vi "AppenderConfigFromDTO.vi"(8 "error in (no error)":errorcluster, 11 "AppenderConfigDTO":T6={"id"="", "threshold"="INFO", "filter"={"mode"="Mirror", "levelMin"="INFO", "levelMax"="INFO", "tagPrefix"=""}, "queueBound"=0, "dropPolicy"="DropOldest", "useUTC"=FALSE}) -> (0 "error out":errorcluster, 3 "AppenderConfig":T1={"id"="", "threshold"=enum."INFO", "filter"={"mode"=enum."Mirror", "levelMin"=enum."INFO", "levelMax"=enum."INFO", "tagPrefix"=""}, "queueBound"=0, "dropPolicy"=enum."DropOldest", "useUTC"=FALSE})   [LabVIEW 2026, in "Lumberjack.lvlib"]
uses:
  Lumberjack.lvlib
  TypeDefs/ConfigDTO/AppenderConfigDTO.ctl
  TypeDefs/ConfigDTO/FilterDTO.ctl
  TypeDefs/AppenderConfig.ctl
  TypeDefs/Severity.ctl
  TypeDefs/Filter.ctl
  TypeDefs/FilterMode.ctl
  TypeDefs/DropPolicy.ctl
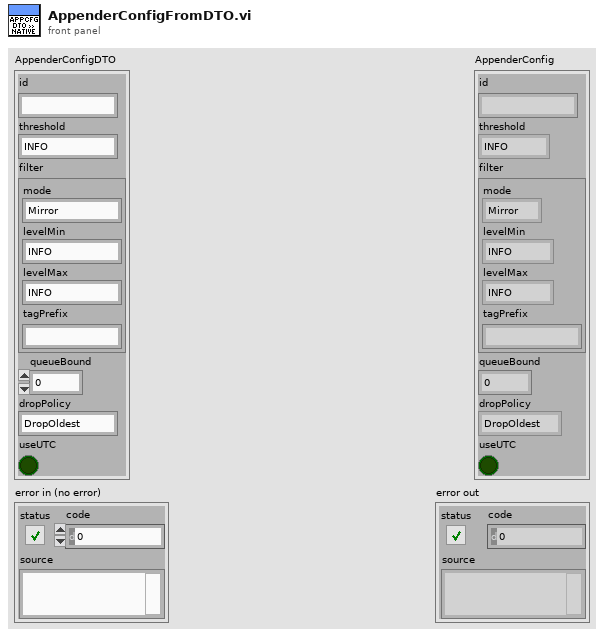
[diagram p1: front panel]
types:
  T1 = typedef "Lumberjack.lvlib/AppenderConfig.ctl" = cluster{"id":string, "threshold":T2, "filter":T3, "queueBound":i32, "dropPolicy":T5, "useUTC":bool}
  T2 = typedef "Lumberjack.lvlib/Severity.ctl" = enum16{"OFF", "FATAL", "ERROR", "WARN", "INFO", "DEBUG", "TRACE", "ALL"}
  T3 = typedef "Lumberjack.lvlib/Filter.ctl" = cluster{"mode":T4, "levelMin":T2, "levelMax":T2, "tagPrefix":string}
  T4 = typedef "Lumberjack.lvlib/FilterMode.ctl" = enum16{"Mirror", "Routed"}
  T5 = typedef "Lumberjack.lvlib/DropPolicy.ctl" = enum16{"DropOldest", "DropNewest", "LevelAware"}
  T6 = typedef "Lumberjack.lvlib/AppenderConfigDTO.ctl" = cluster{"id":string, "threshold":string, "filter":T7, "queueBound":i32, "dropPolicy":string, "useUTC":bool}
  T7 = typedef "Lumberjack.lvlib/FilterDTO.ctl" = cluster{"mode":string, "levelMin":string, "levelMax":string, "tagPrefix":string}
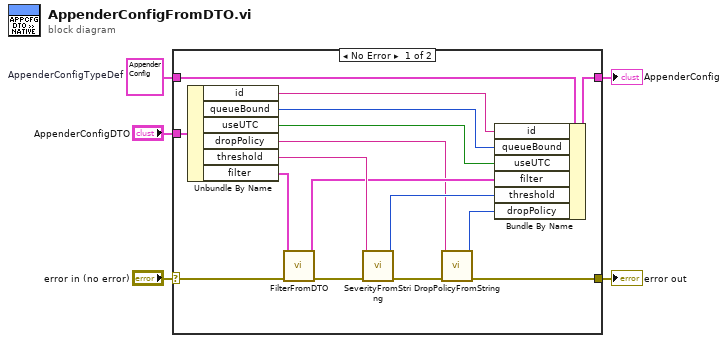
[diagram p0: block diagram]
diagram:
  w2 = T1 {"id"="", "threshold"=enum."INFO", "filter"={"mode"=enum."Mirror", "levelMin"=enum."INFO", "levelMax"=enum."INFO", "tagPrefix"=""}, "queueBound"=0, "dropPolicy"=enum."DropOldest", "useUTC"=FALSE}  # AppenderConfigTypeDef
  n1 = case shown="No Error" "error in (no error)" {
    selector: "error in (no error)" -> [w21 w23]
    tunnel: [w18 w23] -> w4
    tunnel: "AppenderConfigDTO" -> [w16 _]
    tunnel: w2 -> [w15 w22]
    tunnel: [w17 w22] -> w3
    frame No Error {
      n2 = Unbundle By Name(w16) -> ("id"=w14:string, "queueBound"=w13:i32, "useUTC"=w6:bool, "dropPolicy"=w7:string, "threshold"=w11:string, "filter"=w12:T7)
      n3 = call "FilterFromDTO.vi"("error in (no error)"=w21, "FilterDTO"=w12) -> ("error out"=w20:errorcluster, "Filter"=w8:T3)  [unwired: 8 in]
      n4 = call "SeverityFromString.vi"("error in (no error)"=w20, "SeverityString"=w11) -> ("error out"=w19:errorcluster, "Severity"=w10:T2)  [unwired: 8 in]
      n5 = call "DropPolicyFromString.vi"("error in (no error)"=w19, "DropPolicyString"=w7) -> ("error out"=w18:errorcluster, "DropPolicy"=w9:T5)  [unwired: 8 in]
      n6 = Bundle By Name(cluster=w15, "id"=w14, "queueBound"=w13, "useUTC"=w6, "filter"=w8, "threshold"=w10, "dropPolicy"=w9) -> (w17:T1)
    }
    frame Error {
    }
  }
  "AppenderConfig" <- w3
  "error out" <- w4
